vi "read_params.vi"(8 "error in (no error)":errorcluster, 11 "SVR in":refnum<class "SVR.lvclass">) -> (0 "error out":errorcluster, 2 "params":T1={"kernel"="rbf", "degree"=0.0, "gamma"={"gamma_type"="scale", "gamma_float"=0.001}, "coef0"=0.0, "tol"=0.001, "C"=1.0, "epsilon"=0.1, "shrinking"=TRUE, "cache_size"=200.0, "verbose"=FALSE, "max_iter"=-1.0}, 3 "SVR out":refnum<class "SVR.lvclass">)   [LabVIEW 2020, in "SVR.lvclass"]
uses:
  SVR.lvclass
  Controls/svr_params.ctl
  SVR.lvclass/SVR.ctl
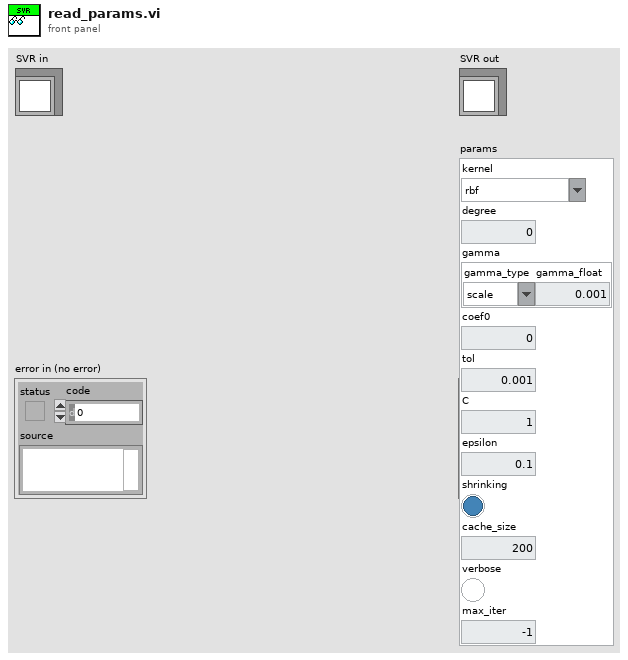
[diagram p1: front panel]
types:
  T1 = typedef "svr_params.ctl" = cluster{"kernel":string, "degree":dbl, "gamma":cluster{"gamma_type":string, "gamma_float":dbl}, "coef0":dbl, "tol":dbl, "C":dbl, "epsilon":dbl, "shrinking":bool, "cache_size":dbl, "verbose":bool, "max_iter":dbl}
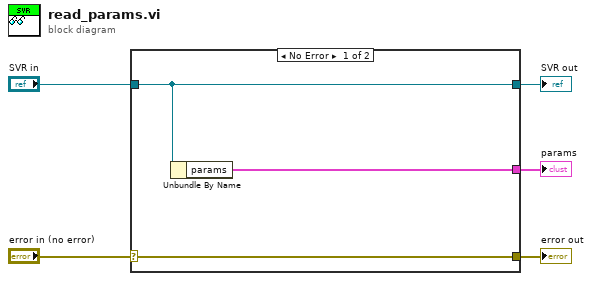
[diagram p0: block diagram]
diagram:
  n1 = case shown="No Error" "error in (no error)" {
    selector: "error in (no error)" -> [w8 w9]
    tunnel: [w8 w9] -> w4
    tunnel: [w7 w10] -> w2
    tunnel: "SVR in" -> [w7 w10]
    tunnel: [w6 _] -> w1
    frame No Error {
      n2 = Unbundle By Name(w7) -> ("params"=w6:T1)
    }
    frame Error {
    }
  }
  "error out" <- w4
  "SVR out" <- w2
  "params" <- w1
